vi "generate_DAC_voltages_V2_subvipackaged.vi"(7 "focus mode?":bool, 8 "derived values":T1, 9 "scan specification":T4={"x amplitude"=0, "x resolution (pixels)"=0, "x offset fly-forward (iterations)"=0, "x offset fly-back (iterations)"=0, "y resolution (nr. of lines)"=0, "y step size"=0, "iterations per pixel"=0, "number of frames"=0, "y offset (pixels)"=0, "number of y-brake lines  (before y-fly-back)"=0, "number y-brake lines (after y-fly-back)"=0, "number of y-fly-back steps"=8, "lines per z step"=0, "number of z/intensity tuples"=0, "number of repetitions (volumes or planes)"=0, "z step size derived"=0, "choose the beginning of z scan"=FALSE, "number of frames (settings)"=0, "FPGA trajectory?"=FALSE}, 10 "counter cluster in":T2, 11 "resonant trigger":bool) -> (0 "acquire?":bool, 1 "fly-back acquisition phase?":bool, 2 "counter cluster out":T2, 3 "DAC voltages":T3 {"ch6" max=4095 step=1; "ch5" max=4095 step=1; "ch4" max=4095 step=1; "ch3" max=4095 step=1; "ch2" max=4095 step=1; "ch1" max=4095 step=1; "ch0" max=4095 step=1})   [LabVIEW 2010]
uses:
  scan_specification_cluster.ctl
  common_typedefs/DAC_voltage_cluster.ctl
  counter_cluster.ctl
  derived_values_cluster.ctl
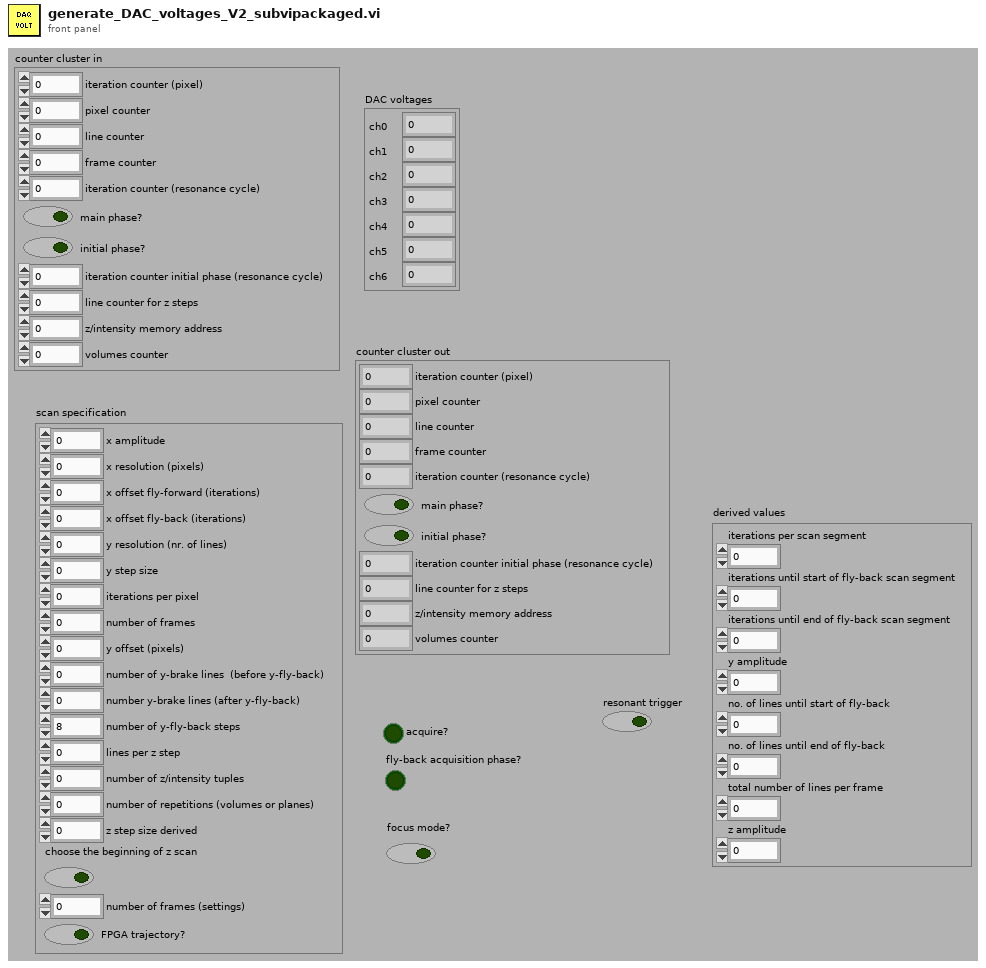
[diagram p1: front panel]
types:
  T1 = typedef "derived_values_cluster.ctl" = cluster{"iterations per scan segment":u16, "iterations until start of fly-back scan segment":u16, "iterations until end of fly-back scan segment":u16, "y amplitude":u16, "no. of lines until start of fly-back":u16, "no. of lines until end of fly-back":u16, "total number of lines per frame ":u16, "z amplitude":u16}
  T2 = typedef "counter_cluster.ctl" = cluster{"iteration counter (pixel)":u16, "pixel counter":u16, "line counter":u16, "frame counter":u16, "iteration counter (resonance cycle)":u16, "main phase?":bool, "initial phase?":bool, "iteration counter initial phase (resonance cycle)":u16, "line counter for z steps":u16, "z/intensity memory address":u32, "volumes counter":u16}
  T3 = typedef "DAC_voltage_cluster.ctl" = cluster{"ch0":u16, "ch1":i16, "ch2":i16, "ch3":u16, "ch4":u16, "ch5":u16, "ch6":u16}
  T4 = typedef "scan_specification_cluster.ctl" = cluster{"x amplitude":u16, "x resolution (pixels)":u16, "x offset fly-forward (iterations)":u16, "x offset fly-back (iterations)":u16, "y resolution (nr. of lines)":u16, "y step size":u16, "iterations per pixel":u16, "number of frames":i32, "y offset (pixels)":u16, "number of y-brake lines  (before y-fly-back)":u16, "number y-brake lines (after y-fly-back)":u16, "number of y-fly-back steps":u16, "lines per z step":u16, "number of z/intensity tuples":u16, "number of repetitions (volumes or planes)":i32, "z step size derived":u16, "choose the beginning of z scan":bool, "number of frames (settings)":i32, "FPGA trajectory?":bool}
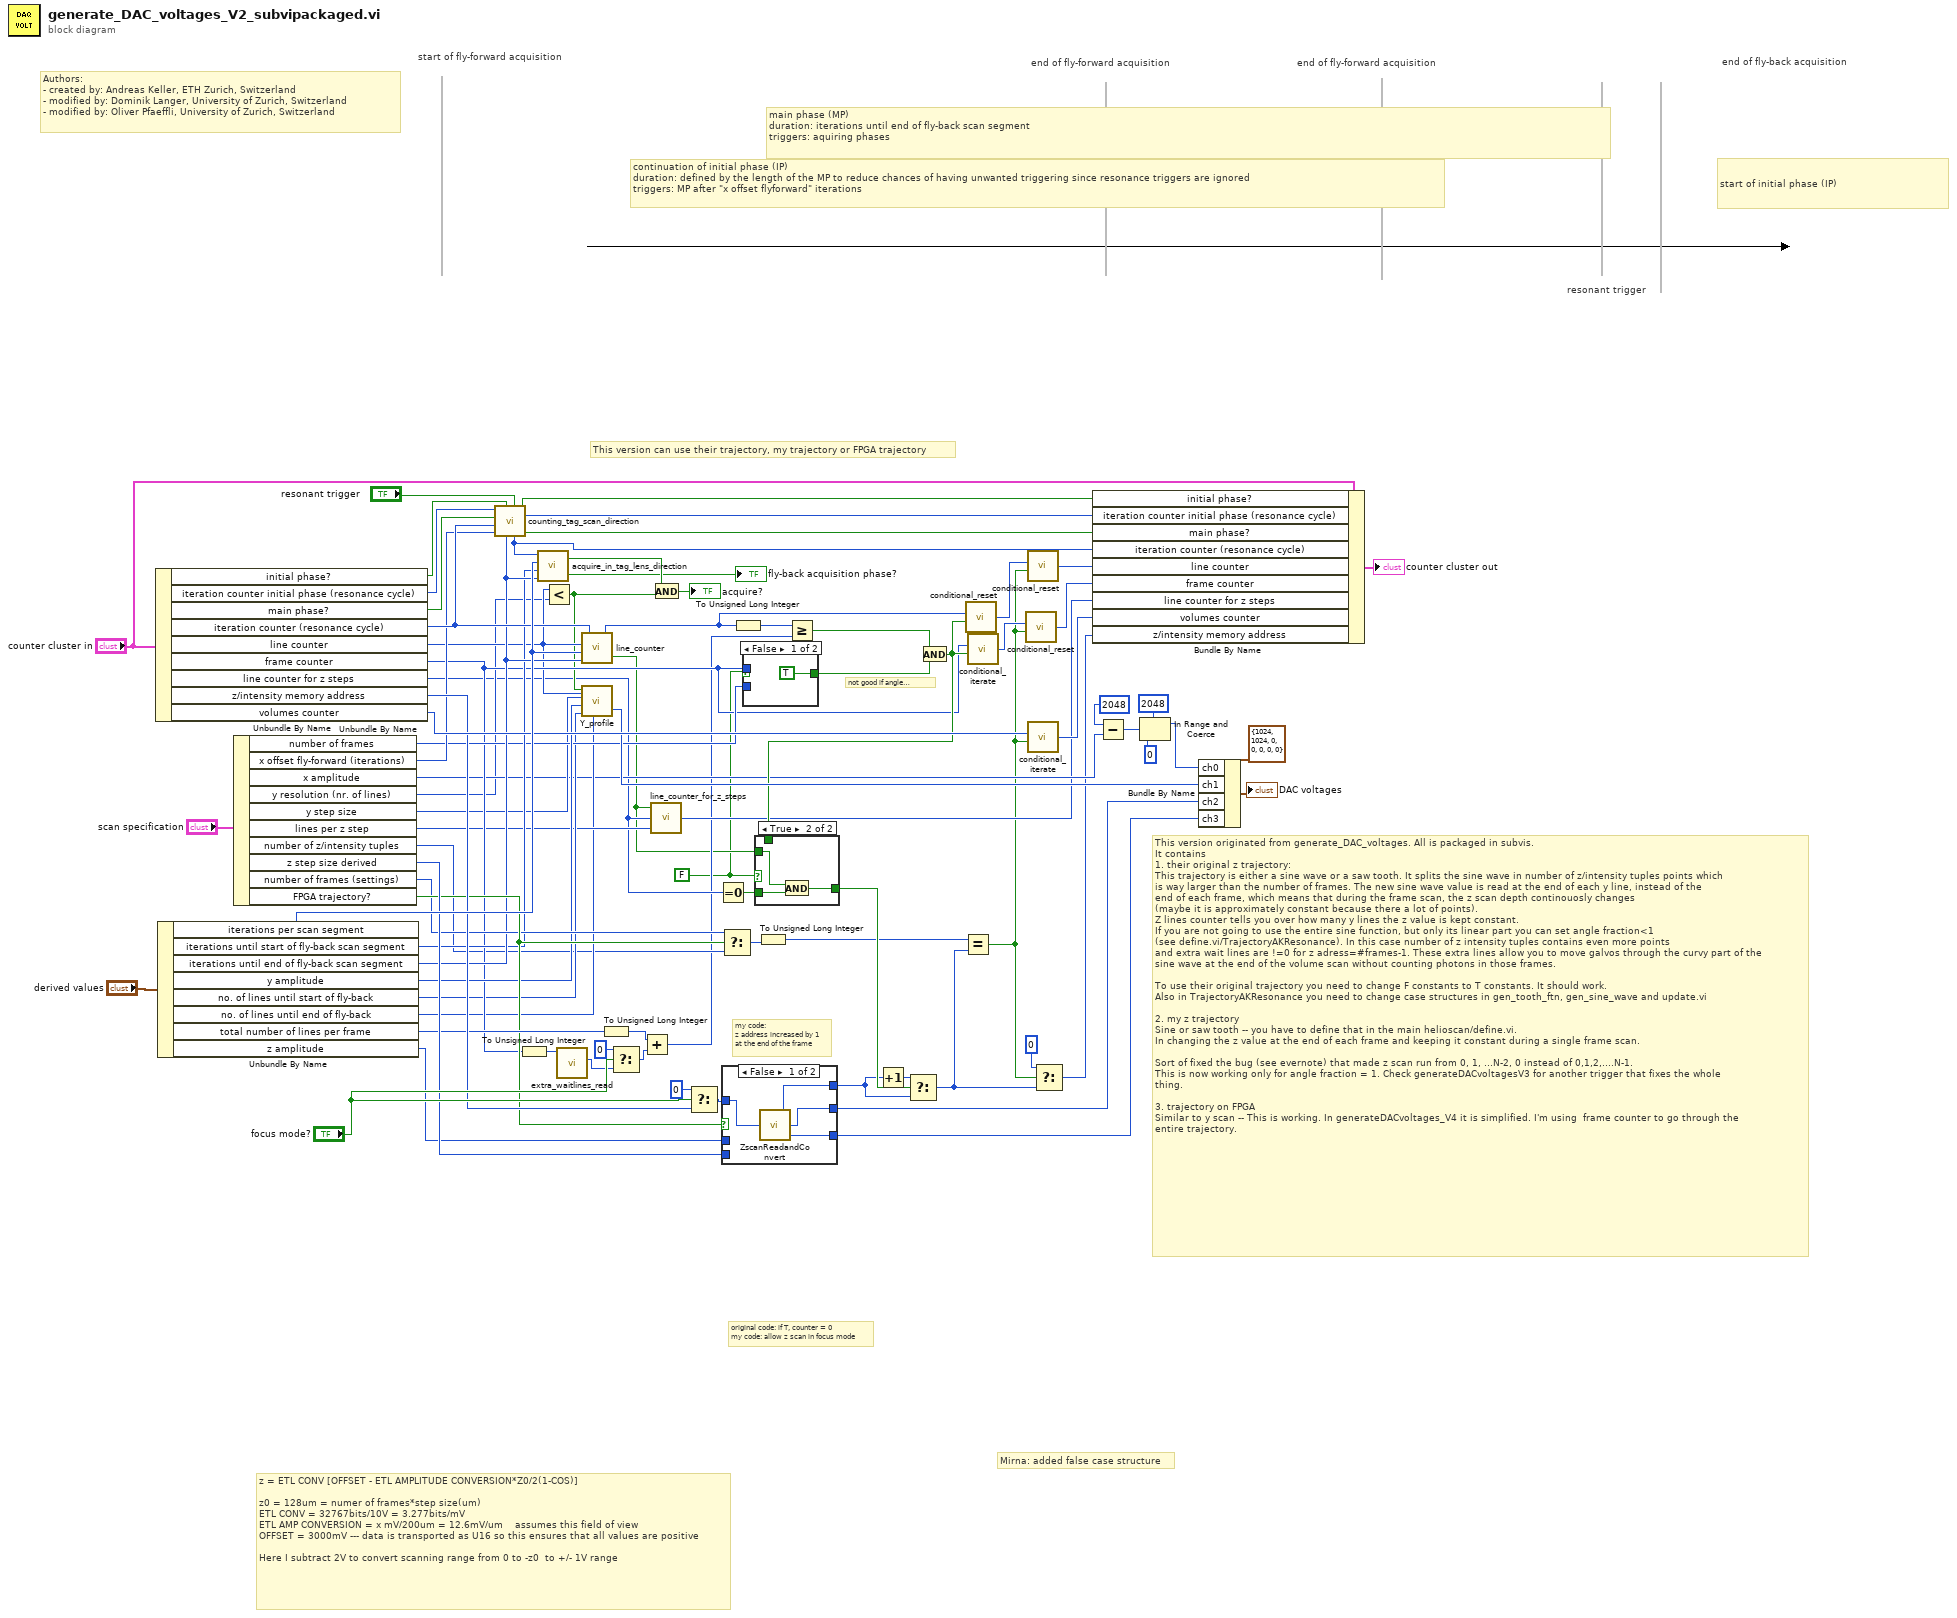
[diagram p0: block diagram]
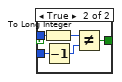
[diagram p2: hidden frame]
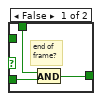
[diagram p3: hidden frame]
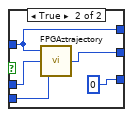
[diagram p4: hidden frame]
diagram:
  w1 = FALSE
  # "not good if angle fraction<1"
  # "This version can use their trajectory, my trajectory or FPGA trajectory"
  # "This version originated from generate_DAC_voltages. All is packaged in subvis. \nIt contains \n1. their original z trajectory:\nThis trajectory is either a sine wave or a saw tooth. It splits the sine wave in number of z/intensity tuples points which\nis way larger than the number of frames. The new sine wave value is read at the end of each y line, instead of the\nend of each frame, which means that during the frame scan, the z scan depth continouosly changes\n(maybe it is approximately constant because there a lot of points). \nZ lines counter tells you over how many y lines the z value is kept constant.\nIf you are not going to use the entire sine function, but only its linear part you can set angle fraction<1 \n(see define.vi/TrajectoryAKResonance). In this case number of z intensity tuples contains even more points\nand extra wait lines are !=0 for z adress=#frames-1. These extra lines allow you to move galvos through the curvy part of the \nsine wave at the end of the volume scan without counting photons in those frames.\n\nTo use their original trajectory you need to change F constants to T constants. It should work.\nAlso in TrajectoryAKResonance you need to change case structures in gen_tooth_ftn, gen_sine_wave and update.vi\n\n2. my z trajectory\nSine or saw tooth -- you have to define that in the main helioscan/define.vi.\nIn changing the z value at the end of each frame and keeping it constant during a single frame scan. \n\nSort of fixed the bug (see evernote) that made z scan run from 0, 1, ...N-2, 0 instead of 0,1,2,....N-1. \nThis is now working only for angle fraction = 1. Check generateDACvoltagesV3 for another trigger that fixes the whole \nthing. \n\n3. trajectory on FPGA\nSimilar to y scan -- This is working. In generateDACvoltages_V4 it is simplified. I'm using  frame counter to go through the \nentire trajectory."
  # "z = ETL CONV [OFFSET - ETL AMPLITUDE CONVERSION*Z0/2(1-COS)]\n\nz0 = 128um = numer of frames*step size(um)\nETL CONV = 32767bits/10V = 3.277bits/mV\nETL AMP CONVERSION = x mV/200um = 12.6mV/um    assumes this field of view\nOFFSET = 3000mV --- data is transported as U16 so this ensures that all values are positive\n\nHere I subtract 2V to convert scanning range from 0 to -z0  to +/- 1V range"
  # "my code:\nz address increased by 1\nat the end of the frame"
  # "original code: if T, counter = 0\nmy code: allow z scan in focus mode"
  # "Mirna: added false case structure"
  # "start of initial phase (IP)"
  # "continuation of initial phase (IP)\nduration: defined by the length of the MP to reduce chances of having unwanted triggering since resonance triggers are ignored\ntriggers: MP after \"x offset flyforward\" iterations"
  # "end of fly-back acquisition"
  # "end of fly-forward acquisition"
  # "end of fly-forward acquisition"
  # "start of fly-forward acquisition"
  # "main phase (MP)\nduration: iterations until end of fly-back scan segment\ntriggers: aquiring phases"
  # "resonant trigger"
  # "Authors: \n- created by: Andreas Keller, ETH Zurich, Switzerland\n- modified by: Dominik Langer, University of Zurich, Switzerland\n- modified by: Oliver Pfaeffli, University of Zurich, Switzerland"
  n1 = Unbundle By Name("counter cluster in") -> ("initial phase?"=w71:bool, "iteration counter initial phase (resonance cycle)"=w34:u16, "main phase?"=w59:bool, "iteration counter (resonance cycle)"=w33:u16, "line counter"=w24:u16, "frame counter"=w25:u16, "line counter for z steps"=w9:u16, "z/intensity memory address"=w54:u32, "volumes counter"=w61:u16)
  n2 = Unbundle By Name("derived values") -> ("iterations per scan segment"=w70:u16, "iterations until start of fly-back scan segment"=w31:u16, "iterations until end of fly-back scan segment"=w32:u16, "y amplitude"=w38:u16, "no. of lines until start of fly-back"=w22:u16, "no. of lines until end of fly-back"=w20:u16, "total number of lines per frame"=w48:u16, "z amplitude"=w39:u16)
  n3 = Unbundle By Name("scan specification") -> ("number of frames"=w26:i32, "x offset fly-forward (iterations)"=w29:u16, "x amplitude"=w18:u16, "y resolution (nr. of lines)"=w12:u16, "y step size"=w23:u16, "lines per z step"=w21:u16, "number of z/intensity tuples"=w14:u16, "z step size derived"=w49:u16, "number of frames (settings)"=w44:i32, "FPGA trajectory?"=w45:bool)
  n4 = call "counting_tag_scan_direction.vi"("resonant trigger"="resonant trigger", "initial phase?"=w71, "iteration counter initial phase (resonance cycle)"=w34, "main phase?"=w59, "iterations until end of fly-back scan segment"=w32, "iteration counter (resonance cycle)"=w33, "x offset fly-forward (iterations)"=w29) -> ("initial phase? OUT"=w36:bool, "iteration counter initial phase (resonance cycle) out"=w35:u16, "main phase? OUT"=w28:bool, "iteration counter (resonance cycle) out"=w4:u16)
  n5 = To Unsigned Long Integer(number=w25) -> (unsigned 32bit integer=w15:u32)
  n6 = call "acquire_in_tag_lens_direction.vi"("iterations until end of fly-back scan segment"=w32, "iterations until start of fly-back scan segment"=w31, "iterations per scan segment"=w70, "iteration counter (resonance cycle) out"=w4) -> ("flyback phase?"=→"fly-back acquisition phase?":bool, "acquire during flyforward or flyback phase?"=w73:bool)
  n7 = Less?(x=w24, y=w12) -> (x < y?=w10:bool)
  n8 = call "extra_waitlines_read.vi"("address extra waitlines IN"=w15) -> ("extra waitline data"=w42:u32)  [unwired: 9 in, 1 out]
  n9 = call "line_counter.vi"("iterations until end of fly-back scan segment"=w32, "iterations per scan segment"=w70, "line counter in"=w24, "iteration counter (resonance cycle)"=w33) -> ("end of line?"=w2:bool, "line counter out"=w13:u16)
  n10 = call "Y_profile.vi"("no. of lines until end of fly-back"=w20, "line counter"=w24, "no. of lines until start of fly-back"=w22, "y amplitude"=w38, "y step size"=w23, "y acquire? (line counter<number of lines)"=w10) -> ("y signal"=w58:i16)  [unwired: 1 in]
  n11 = To Unsigned Long Integer(number=w48) -> (unsigned 32bit integer=w46:u32)
  n12 = Select(t=u32 0, s="focus mode?", f=w42) -> (s? t:f=w63:u32)
  n13 = Add(x=w46, y=w63) -> (x+y=w8:u32)
  n14 = call "line_counter_for_z_steps.vi"("lines per z step"=w21, "line counter for z steps"=w9, "end of line?"=w2) -> ("line counter for z steps out"=w16:u16)
  n15 = And(x=w73, y=w10) -> (x .and. y?=→"acquire?":bool)
  n16 = Select(t=u32 0, s="focus mode?", f=w54) -> (s? t:f=w55:u32)
  n17 = Equal To 0?(x=w9) -> (x = 0?=w68:bool)
  n18 = Select(t=w44, s=w45, f=w14) -> (s? t:f=w53:i32)
  n19 = case shown="False" w45 {
    tunnel: [w84 u16 0 ("intensity")] -> w57
    tunnel: [w86 w87] -> w6
    tunnel: [w83 w90] -> w56
    tunnel: w55 -> [w85 w87]
    tunnel: w49 -> [_ w91]
    tunnel: w39 -> [_ w89]
    frame False {
      n20 = call "ZscanReadandConvert.vi"("z/intensity memory address"=w85) -> ("intensity profile"=w84:u16, "z profile"=w83:u16, "address out"=w86:u32)
    }
    frame True {
      n21 = call "FPGAztrajectory.vi"("z step size derived"=w91, "z amplitude"=w89, "z/intensity memory address"=w87) -> ("Z trajectory"=w90:i16)
    }
  }
  n22 = To Unsigned Long Integer(number=w13) -> (unsigned 32bit integer=w43:u32)
  n23 = case shown="False" w1 {
    tunnel: w26 -> [_ w95]
    tunnel: w25 -> [_ w94]
    tunnel: [TRUE w93] -> w19
    frame False {
    }
    frame True {
      n24 = To Long Integer(number=w94) -> (32bit integer=w96:i32)
      n25 = Decrement(x=w95) -> (x-1=w97:i32)
      n26 = Not Equal?(x=w96, y=w97) -> (x != y?=w93:bool)
    }
  }
  n27 = To Unsigned Long Integer(number=w53) -> (unsigned 32bit integer=w41:u32)
  n28 = Greater Or Equal?(x=w43, y=w8) -> (x >= y?=w64:bool)
  n29 = Increment(x=w6) -> (x+1=w69:u32)
  n30 = And(x=w64, y=w19) -> (x .and. y?=w50:bool)
  n31 = case shown="True" w1 {
    tunnel: w68 -> [w100 w103]
    tunnel: w2 -> [_ w102]
    tunnel: [w99 w101] -> w47
    tunnel: w50 -> [w98 _]
    frame False {
      # "end of\nframe?"
      n32 = And(x=w98, y=w100) -> (x .and. y?=w99:bool)
    }
    frame True {
      n33 = And(x=w102, y=w103) -> (x .and. y?=w101:bool)
    }
  }
  n34 = Select(t=w69, s=w47, f=w6) -> (s? t:f=w5:u32)
  n35 = Equal?(x=w41, y=w5) -> (x = y?=w3:bool)
  n36 = call "conditional_reset.vi"("reset?"=w50, "number in"=w13) -> ("number out"=w66:u16)  [unwired: 4 in]
  n37 = call "conditional_iterate.vi"("iterate?"=w50, "number in"=w25) -> ("number out"=w51:u16)  [unwired: 4 in]
  n38 = call "conditional_reset.vi"("reset?"=w3, "number in"=w51) -> ("number out"=w52:u16)  [unwired: 4 in]
  n39 = call "conditional_reset.vi"("reset?"=w3, "number in"=w66) -> ("number out"=w65:u16)  [unwired: 4 in]
  n40 = call "conditional_iterate.vi"("iterate?"=w3, "number in"=w61) -> ("number out"=w67:u16)  [unwired: 4 in]
  n41 = Select(t=u32 0, s=w3, f=w5) -> (s? t:f=w7:u32)
  n42 = Bundle By Name(cluster="counter cluster in", "initial phase?"=w36, "iteration counter initial phase (resonance cycle)"=w35, "main phase?"=w28, "iteration counter (resonance cycle)"=w4, "line counter"=w65, "frame counter"=w52, "line counter for z steps"=w16, "volumes counter"=w67, "z/intensity memory address"=w7) -> (→"counter cluster out":T2)
  n43 = Subtract(x=u16 2048, y=w18) -> (x-y=w77:u16)
  n44 = In Range and Coerce(upper limit=u16 2048, x=w77, lower limit=u16 0) -> (coerced(x)=w76:u16)  [unwired: 1 out]
  n45 = Bundle By Name(cluster=T3 {"ch0"=1024, "ch1"=1024, "ch2"=0, "ch3"=0, "ch4"=0, "ch5"=0, "ch6"=0} ("DAC voltage"), "ch0"=w76, "ch1"=w58, "ch2"=w56, "ch3"=w57) -> (→"DAC voltages":T3)
